vi "PS FPGA IIR Filter Core.vi"(0 "input data":fxp<+/-,20,5>, 1 "coeff_a":fxp<+/-,20,2>[](array[numeric])=[0.0, 0.0, 0.0], 2 "coeff_b":fxp<+/-,20,2>[](array[numeric])=[1.0, 0.0, 0.0], 9 "input valid":bool, 12 "reset":bool) -> (4 "output data":fxp<+/-,20,5> format="%.31g", 10 "output valid":bool, 14 "ready for input":bool)   [LabVIEW 2011]
doc: "----------------------\n\nThis filter is configured as follows:\n\n<b>Filter Configuration</b>\nType: Single Rate\nStructure: IIR Cascaded Second-Order Sections Form II Transposed\n\n<b>Input Data Type</b>\nType: fixed-point <±,20,5> [-1.600000E+1,1.599997E+1]:3.051758E-5\n\n<b>Output Data Type</b>\nType: fixed-point <±,20,5> [-1.600000E+1,1.599997E+1]:3.051758E-5\nRounding mode: Truncate\nOverflow mode: Wrap\n\n<b>Implementation</b>\nNumber of channels: 8\nMaximum input sampling rate per channel @ 40MHz: 1.667MHz\nGain processing: On Host\nMethod: Multiply-Accumulate\n\n<b>Execution Mode</b>\nInside single-cycle Timed Loop\nThroughput: 3 cycles/sample\n\n<b>Estimated Resources</b>\n2 20x32 multiplier"
uses:
  <vilib>/rvi/FXPMathLib/FxpMul/XNode/nifxpmath_Multiplier.xnode
  <vilib>/rvi/FXPMathLib/basic elements/FxpDiscreteDelay/XNode/nifxpmath_DiscreteDelay.xnode
  <vilib>/rvi/FXPMathLib/sim/FxpSim.dll
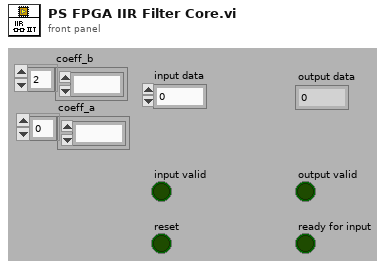
[diagram p1: front panel]
types:
  T1 = cluster{"update  v?":bool, "write s1?":bool, "init?":bool}
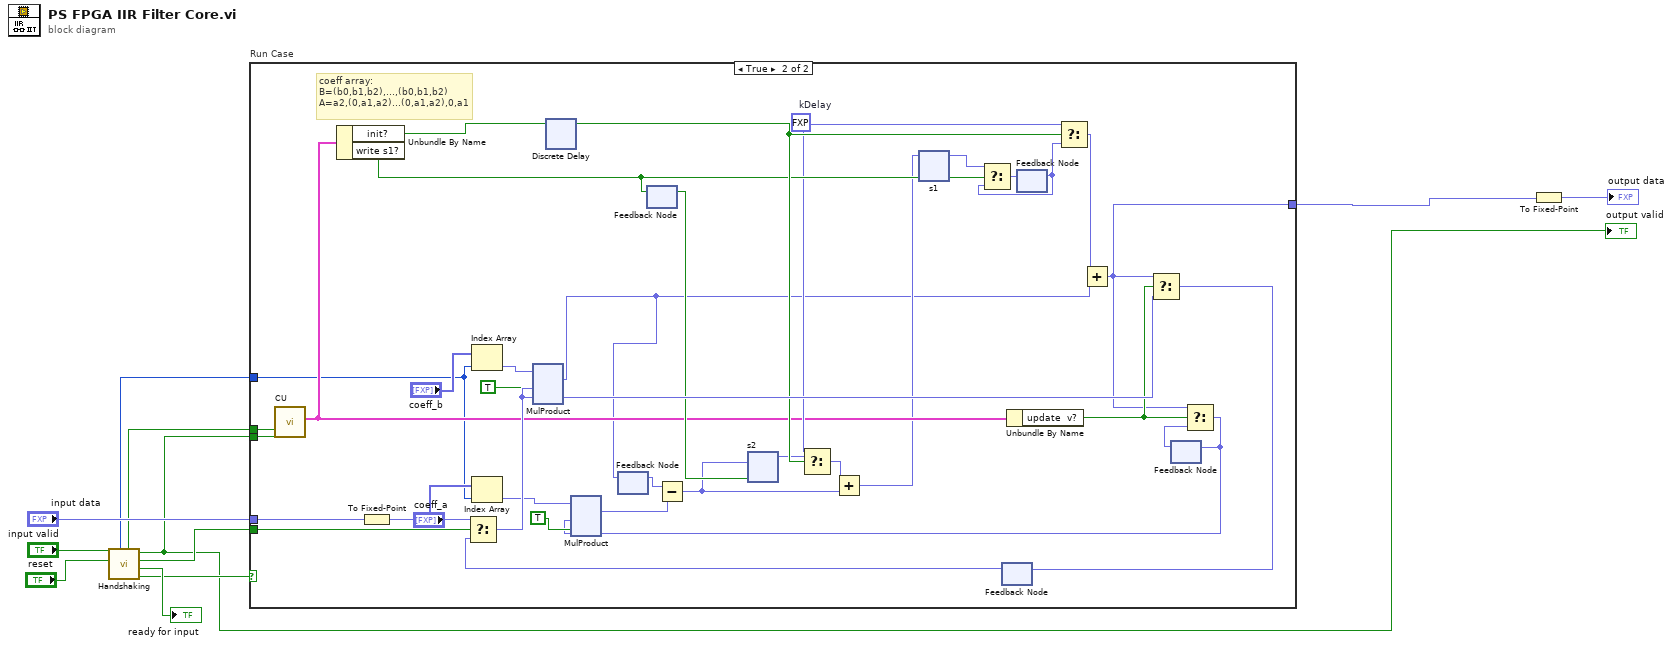
[diagram p0: block diagram]
diagram:
  n1 = call "Handshaking"("reset"="reset", "input valid"="input valid") -> ("run?"=w8:bool, "ready for input"=→"ready for input":bool, "load"=w4:bool, "output valid"=w1:bool, "reset for cu"=w7:bool, "idx"=w5:i16)  [unwired: 4 out]
  "output valid" <- w1
  n2 = case "Run Case" shown="True" w8 {
    tunnel: "input data" -> [_ w12]
    tunnel: w1 -> [_ w37]
    tunnel: w4 -> [_ w13]
    tunnel: w7 -> [_ w36]
    tunnel: w5 -> [_ w15]
    tunnel: [_ w16] -> w2
    frame False {
    }
    frame True {
      w22 = fxp<+/-,32,6> 0.0  # kDelay
      # "coeff array:\nB=(b0,b1,b2),...,(b0,b1,b2)\nA=a2,(0,a1,a2)...(0,a1,a2),0,a1"
      n3 = call "CU"("output valid"=w37, "global reset"=w36) -> ("Control signal"=w21:T1)  [unwired: 9 out]
      n4 = Unbundle By Name(w21) -> ("init?"=w35:bool, "write s1?"=w23:bool)
      n5 = To Fixed-Point ("toMultiplicand")(number=w12) -> (fixed-point=w43:fxp<+/-,32,6>)  [unwired: 1 out]
      n6 = Index Array(array="coeff_b", index=w15) -> (element=w42:fxp<+/-,20,2>)
      n7 = Index Array(array="coeff_a", index=w15) -> (element=w24:fxp<+/-,20,2>)
      n8 = xnode ("Discrete Delay")("D"=w35) -> ("Q"=w33:bool)
      n9 = feedback #1() -> (w29:fxp<+/-,32,6>)  [unwired: 1 out]
      n10 = feedback-in #2(w23) -> ()
      n11 = feedback #2() -> (w31:bool)  [unwired: 1 out]
      n12 = feedback #3() -> (w39:fxp<+/-,32,6>)  [unwired: 1 out]
      n13 = Select(t=w43, s=w13, f=w39) -> (s? t:f=w41:fxp<+/-,32,6>)
      n14 = xnode "MulProduct"("x"=w42, "y"=w41, "input valid"=TRUE) -> ("x*y"=w14:fxp<+/-,32,6>)  [unwired: 1 in, 2 out]
      n15 = feedback-in #1(w14) -> ()
      n16 = Unbundle By Name(w21) -> ("update  v?"=w38:bool)
      n17 = feedback #4() -> (w26:fxp<+/-,32,6>)  [unwired: 1 out]
      n18 = Select(t=w22, s=w33, f=w26) -> (s? t:f=w40:fxp<+/-,32,6>)
      n19 = Add ("AddSum")(x=w40, y=w14) -> (x+y=w16:fxp<+/-,32,6>)
      n20 = Select(t=w16, s=w38, f=w41) -> (s? t:f=w18:fxp<+/-,32,6>)
      n21 = feedback-in #3(w18) -> ()
      n22 = feedback #5() -> (w30:fxp<+/-,32,6>)  [unwired: 1 out]
      n23 = Select(t=w16, s=w38, f=w30) -> (s? t:f=w17:fxp<+/-,32,6>)
      n24 = xnode "MulProduct"("x"=w24, "y"=w17, "input valid"=TRUE) -> ("x*y"=w44:fxp<+/-,32,6>)  [unwired: 1 in, 2 out]
      n25 = Subtract ("SubSum")(x=w29, y=w44) -> (x-y=w19:fxp<+/-,32,6>)
      n26 = xnode ("s2")("D"=w19, "enable"=w31) -> ("Q"=w32:fxp<+/-,32,6>)
      n27 = Select(t=w22, s=w33, f=w32) -> (s? t:f=w34:fxp<+/-,32,6>)
      n28 = Add ("AddSum")(x=w34, y=w19) -> (x+y=w20:fxp<+/-,32,6>)
      n29 = xnode ("s1")("D"=w20, "enable"=w23) -> ("Q"=w28:fxp<+/-,32,6>)
      n30 = Select(t=w28, s=w23, f=w26) -> (s? t:f=w27:fxp<+/-,32,6>)
      n31 = feedback-in #4(w27) -> ()
      n32 = feedback-in #5(w17) -> ()
    }
  }
  n33 = To Fixed-Point ("toOutput")(number=w2) -> (fixed-point=→"output data":fxp<+/-,20,5>)  [unwired: 1 out]
